vi "Pause.vi"(8 "error in (no error)":errorcluster, 11 "State in":T1={"State"=enum."Idle", "Start Time"=timestamp(0 s since 1904-01-01), "Configuration"={"Cycle Period"=0.0, "Manual Entry"=0.0, "Output Device"=enum."Default", "EPOS4 Settings"={"VISA resource name"="", "axis"={"keyHandle"=1, "nodeId"=1}, "Simulated?"=FALSE}}, "Current Time"=timestamp(0 s since 1904-01-01), "First Iteration"=FALSE, "Data"={"Centrifuge Speed"=0.0}, "Process Name"="", "Centrifuge On?"=enum."Off", "Output Error"=FALSE, "Log Started"=FALSE}) -> (0 "error out":errorcluster, 3 "State out":T1={"State"=enum."Idle", "Start Time"=timestamp(0 s since 1904-01-01), "Configuration"={"Cycle Period"=0.0, "Manual Entry"=0.0, "Output Device"=enum."Default", "EPOS4 Settings"={"VISA resource name"="", "axis"={"keyHandle"=1, "nodeId"=1}, "Simulated?"=FALSE}}, "Current Time"=timestamp(0 s since 1904-01-01), "First Iteration"=FALSE, "Data"={"Centrifuge Speed"=0.0}, "Process Name"="", "Centrifuge On?"=enum."Off", "Output Error"=FALSE, "Log Started"=FALSE})   [LabVIEW 2018, in "Centrifuge Module.lvlib" / "Centrifuge Module Engine.lvlib"]
uses:
  Centrifuge Module Engine.lvlib
  State Cluster.ctl
  State Enum.ctl
  Centrifuge Module Settings Cluster.ctl
  EPOS4/Controls/Device Selection.ctl
  EPOS4/Controls/EPOS Communication Settings.ctl
  Tag VIs/Tag FGV Operation Enum.ctl
  Shared Variables/Dynamic Shared Variables.lvlib
  EPOS4/EPOS4.lvlib
  Centrifuge Module.lvlib
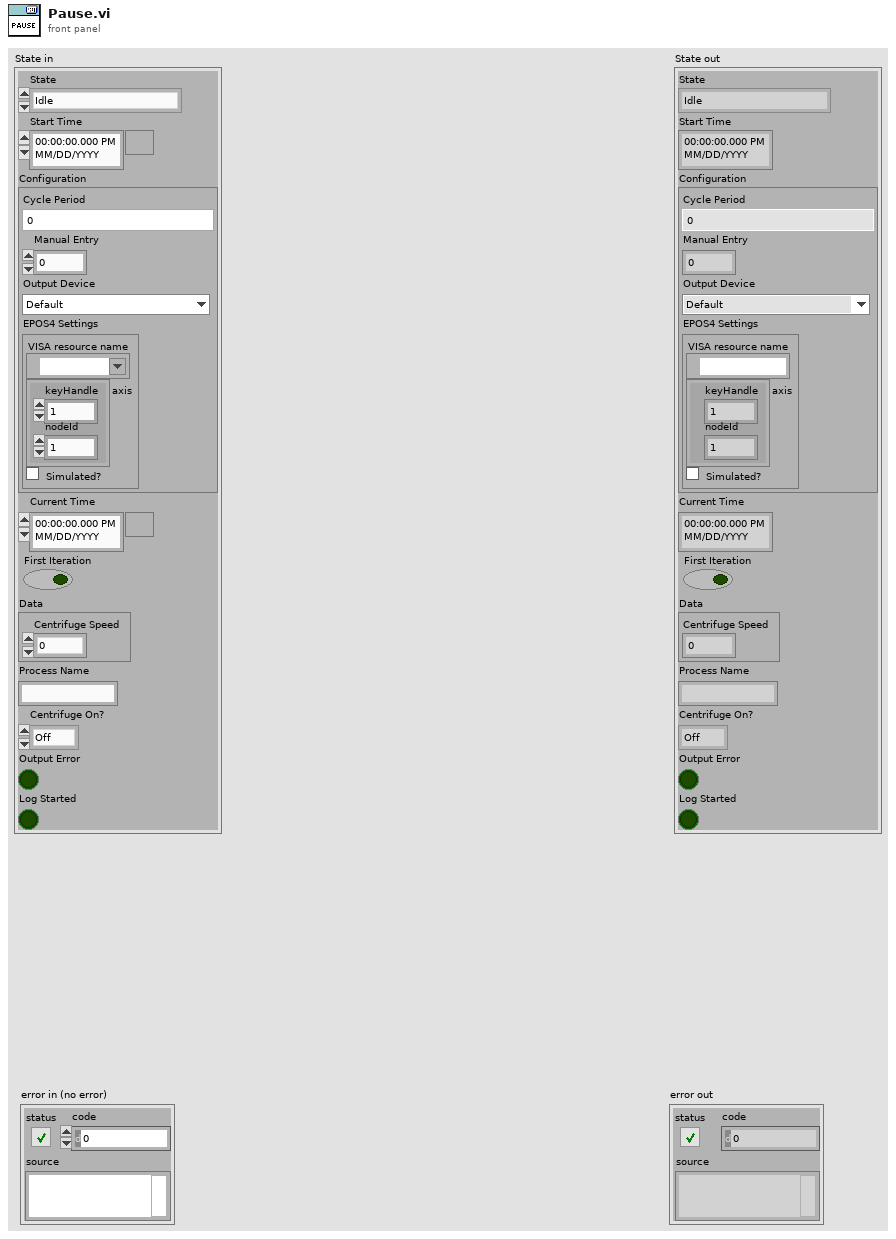
[diagram p1: front panel]
types:
  T1 = typedef "Centrifuge Module.lvlib/Centrifuge Module Engine.lvlib/State Cluster.ctl" = cluster{"State":T2, "Start Time":timestamp, "Configuration":T3, "Current Time":timestamp, "First Iteration":bool, "Data":cluster{"Centrifuge Speed":dbl}, "Process Name":string, "Centrifuge On?":enum16{"Off", "On", "Not Initialized"}, "Output Error":bool, "Log Started":bool}
  T2 = typedef "Centrifuge Module.lvlib/Centrifuge Module Engine.lvlib/State Enum.ctl" = enum16{"Measuring", "Idle", "Paused"}
  T3 = typedef "Centrifuge Module.lvlib/Centrifuge Module Settings Cluster.ctl" = cluster{"Cycle Period":dbl, "Manual Entry":dbl, "Output Device":T4, "EPOS4 Settings":T5}
  T4 = typedef "Device Selection.ctl" = enum16{"Default", "EPOS4"}
  T5 = typedef "EPOS4.lvlib/EPOS Communication Settings.ctl" = cluster{"VISA resource name":refnum<visa-resource-name>, "axis":cluster{"keyHandle":u32, "nodeId":u16}, "Simulated?":bool}
  T6 = typedef "Centrifuge Module.lvlib/Centrifuge Module Tag Names Cluster.ctl" = cluster{"Centrifuge Speed":string, "Output Device Tag":string}
  T7 = typedef "Tag FGV Operation Enum.ctl" = enum16{"Init", "Set Notification Queue", "Create Tag", "Commit", "Write Tag (Numeric)", "Write Tag (Boolean)", "Read All Tags", "Read One Tag", "Delete Tag Category", "Set Alarm Parameters (Numeric)", "Set Alarm Parameters (Boolean)", "Enable All Alarms", "Disable All Alarms", "Delete All Tags", "Read Alarms", "Ack Alarm", "Read Alarm Parameters (Numeric)", "Read Alarm Parameters (Boolean)"}
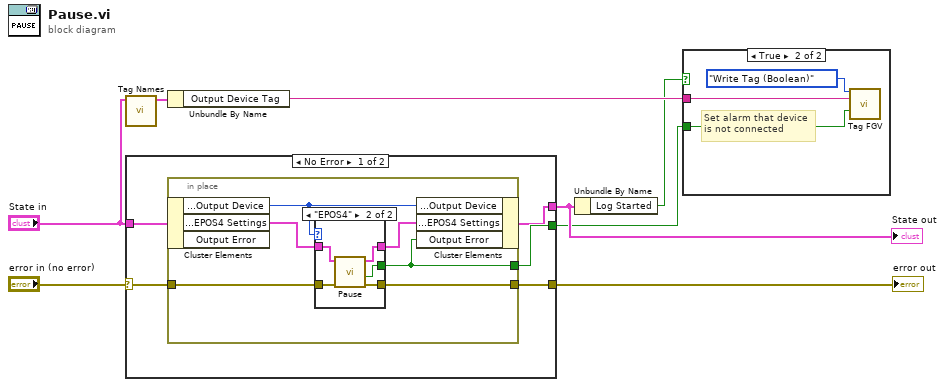
[diagram p0: block diagram]
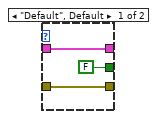
[diagram p3: hidden frame]
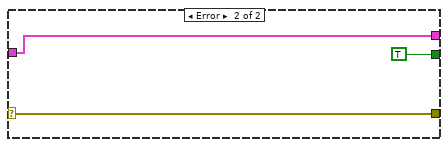
[diagram p4: hidden frame]
diagram:
  n1 = call "Tag Names.vi"("State In"="State in") -> ("Centrifuge Module Tag Names"=w5:T6)  [unwired: 8 in, 2 out]
  n2 = case shown="No Error" "error in (no error)" {
    selector: "error in (no error)" -> [w12 w30]
    tunnel: [w13 w30] -> w7
    tunnel: "State in" -> [w10 w29]
    tunnel: [w9 w29] -> w2
    tunnel: [w11 TRUE ("Connection Error")] -> w1
    frame No Error {
      n3 = in-place {
        in-place-border: [w18] -> w13
        in-place-border: w12 -> [w19]
        in-place-border: [w17] -> w11
        n4 = in-place-cluster #1(w10) -> ("Configuration.Output Device"=w14:T4, "Configuration.EPOS4 Settings"=w15:T5)  [unwired: 1 out]
        n5 = case shown="\"EPOS4\"" w14 {
          tunnel: w19 -> [w22 w27]
          tunnel: [w22 w26] -> w18
          tunnel: [FALSE ("Connection Error") w25] -> w17
          tunnel: [w20 w24] -> w16
          tunnel: w15 -> [w20 w23]
          frame "Default", Default {
          }
          frame "EPOS4" {
            n6 = call "Pause.vi"("error in (no error)"=w27, "EPOS4 Settings in"=w23) -> ("error out"=w26:errorcluster, "Connection Error"=w25:bool, "EPOS4 Settings out"=w24:T5)  [unwired: 7 in]
          }
        }
        n7 = in-place-cluster #1("Configuration.Output Device"=w14, "Configuration.EPOS4 Settings"=w16, "Output Error"=w17) -> (w9:T1)
      }
    }
    frame Error {
    }
  }
  "error out" <- w7
  "State out" <- w2
  n8 = Unbundle By Name(w5) -> ("Output Device Tag"=w6:string)
  n9 = Unbundle By Name(w2) -> ("Log Started"=w4:bool)
  n10 = case shown="True" w4 {
    tunnel: w6 -> [_ w32]
    tunnel: w1 -> [_ w31]
    frame False {
    }
    frame True {
      # "Set alarm that device\nis not connected"
      n11 = call "Tag FGV.vi"("Operation"=Tag_FGV_Operation_Enum."Write Tag (Boolean)", "Tag Name"=w32, "Data"=w31) -> ()  [unwired: 5 in, 8 out]
    }
  }
